vi "UA to DCAF DataType.vi"(1 "OPC UA Data Type":T1 items=["Boolean"=1, "SByte"=2, "Byte"=3, "Int16"=4, "UInt16"=5, "Int32"=6, "UInt32"=7, "Int64"=8, "UInt64"=9, "Float"=10, "Double"=11, "String"=12, "DateTime"=13, "ByteString"=15, "Array of Boolean"=101, "Array of SByte"=102, "Array of Byte"=103, "Array of Int16"=104, "Array of UInt16"=105, "Array of Int32"=106, "Array of UInt32"=107, "Array of Int64"=108, "Array of UInt64"=109, "Array of Float"=110, "Array of Double"=111, "Array of String"=112, "Array of DateTime"=113, "Array of ByteString"=115]) -> (0 "DCAF Datatype":T2)   [LabVIEW 2013, in "OPC UA configuration.lvclass"]
doc: "Typecast the OPC UA datatype to one compatible with the DCAF engine"
uses:
  OPC UA configuration.lvclass
  <vilib>/NI/Tag Bus/tag/Data Type.ctl
  OPC UA Data Type.ctl
  <vilib>/NI/Tag Bus/tag/tag descriptor.lvclass
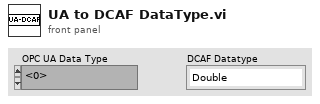
[diagram p1: front panel]
types:
  T1 = typedef "OPC UA configuration.lvclass/OPC UA Data Type.ctl" = u16
  T2 = typedef "tag bus.lvlib/tag descriptor.lvclass/Data Type.ctl" = enum16{"Double", "Single", "I64", "I32", "I16", "I8", "U64", "U32", "U16", "U8", "Boolean", "String", "Array of Double", "Array of Single", "Array of I64", "Array of I32", "Array of I16", "Array of I8", "Array of U64", "Array of U32", "Array of U16", "Array of U8", "Array of Boolean", "Array of String"}
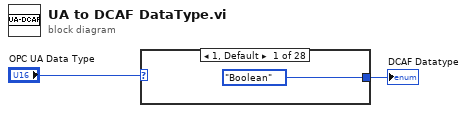
[diagram p0: block diagram]
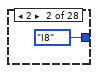
[diagram p2: hidden frame]
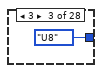
[diagram p3: hidden frame]
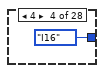
[diagram p4: hidden frame]
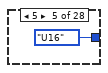
[diagram p5: hidden frame]
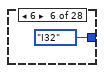
[diagram p6: hidden frame]
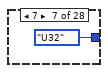
[diagram p7: hidden frame]
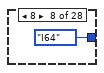
[diagram p8: hidden frame]
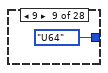
[diagram p9: hidden frame]
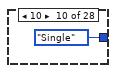
[diagram p10: hidden frame]
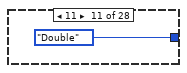
[diagram p11: hidden frame]
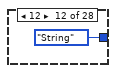
[diagram p12: hidden frame]
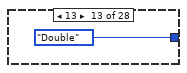
[diagram p13: hidden frame]
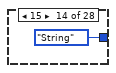
[diagram p14: hidden frame]
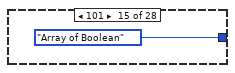
[diagram p15: hidden frame]
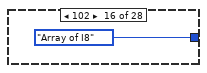
[diagram p16: hidden frame]
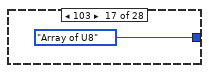
[diagram p17: hidden frame]
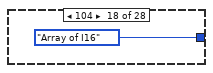
[diagram p18: hidden frame]
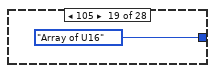
[diagram p19: hidden frame]
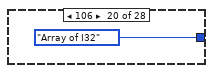
[diagram p20: hidden frame]
diagram:
  n1 = case shown="1, Default" "OPC UA Data Type" {
    tunnel: [Data_Type."Boolean" ("DCAF Datatype") Data_Type."I8" ("DCAF Datatype") Data_Type."U8" ("DCAF Datatype") Data_Type."I16" ("DCAF Datatype") Data_Type."U16" ("DCAF Datatype") Data_Type."I32" ("DCAF Datatype") Data_Type."U32" ("DCAF Datatype") Data_Type."I64" ("DCAF Datatype") Data_Type."U64" ("DCAF Datatype") Data_Type."Single" ("DCAF Datatype") Data_Type."Double" ("DCAF Datatype") Data_Type."String" ("DCAF Datatype") Data_Type."Double" ("DCAF Datatype") Data_Type."String" ("DCAF Datatype") Data_Type."Array of Boolean" ("DCAF Datatype") Data_Type."Array of I8" ("DCAF Datatype") Data_Type."Array of U8" ("DCAF Datatype") Data_Type."Array of I16" ("DCAF Datatype") Data_Type."Array of U16" ("DCAF Datatype") Data_Type."Array of I32" ("DCAF Datatype") Data_Type."Array of U32" ("DCAF Datatype") Data_Type."Array of I64" ("DCAF Datatype") Data_Type."Array of U64" ("DCAF Datatype") Data_Type."Array of Single" ("DCAF Datatype") Data_Type."Array of Double" ("DCAF Datatype") Data_Type."Array of String" ("DCAF Datatype") Data_Type."Array of Double" ("DCAF Datatype") Data_Type."Array of String" ("DCAF Datatype")] -> w2
    frame 1, Default {
    }
    frame 2 {
    }
    frame 3 {
    }
    frame 4 {
    }
    frame 5 {
    }
    frame 6 {
    }
    frame 7 {
    }
    frame 8 {
    }
    frame 9 {
    }
    frame 10 {
    }
    frame 11 {
    }
    frame 12 {
    }
    frame 13 {
    }
    frame 15 {
    }
    frame 101 {
    }
    frame 102 {
    }
    frame 103 {
    }
    frame 104 {
    }
    frame 105 {
    }
    frame 106 {
    }
    frame 107 {
    }
    frame 108 {
    }
    frame 109 {
    }
    frame 110 {
    }
    frame 111 {
    }
    frame 112 {
    }
    frame 113 {
    }
    frame 115 {
    }
  }
  "DCAF Datatype" <- w2
